vi "Ballard - 1553 - Raw Data Word Channel.vi"(8 "error in (no error)":errorcluster, 11 "Node Ptr":T1 format="%.0x") -> (0 "error out":errorcluster)   [LabVIEW 2017, in "Ballard 1553 System Explorer.lvlib"]
uses:
  Ballard 1553 System Explorer.lvlib
  <vilib>/NI Veristand/Custom Device API/Custom Device Item Ref.ctl
  <vilib>/NI VeriStand/Custom Device API/Custom Device API.lvlib
panel:
  out "Raw Data Default Value":u16 format="%.0x"
  in  "Header":cluster{"Section Name":string}={"Section Name"="Ballard - MIL-STD-1553 - Custom Device - Raw Data Word Channel"}
  in  "Description":string
  in  "Name":string
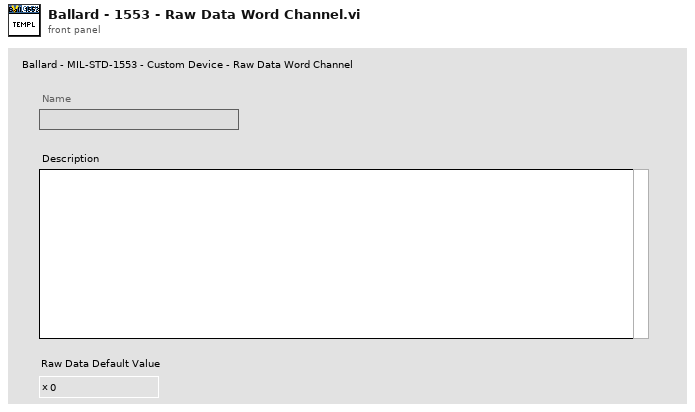
[diagram p1: front panel]
types:
  T1 = typedef "Custom Device API.lvlib/Custom Device Item Ref.ctl" = u64
  T2 = typedef "Custom Device API.lvlib/Custom Device Channel.ctl" = cluster{"Type":T3, "Units":string, "Default Value":dbl, "Faultable":bool, "Scalable":bool}
  T3 = typedef "Custom Device API.lvlib/Custom Device Channel Type.ctl" = enum16{"Input", "Output"}
  T4 = typedef "Custom Device API.lvlib/Custom Device Item Info.ctl" = cluster{"Name":string, "Is Channel":bool, "GUID":string, "Is Waveform":bool}
  T5 = typedef "Custom Device API.lvlib/Custom Device Commands.ctl" = enum16{"Default", "Item renamed", "Shutdown", "Dynamic button pressed"}
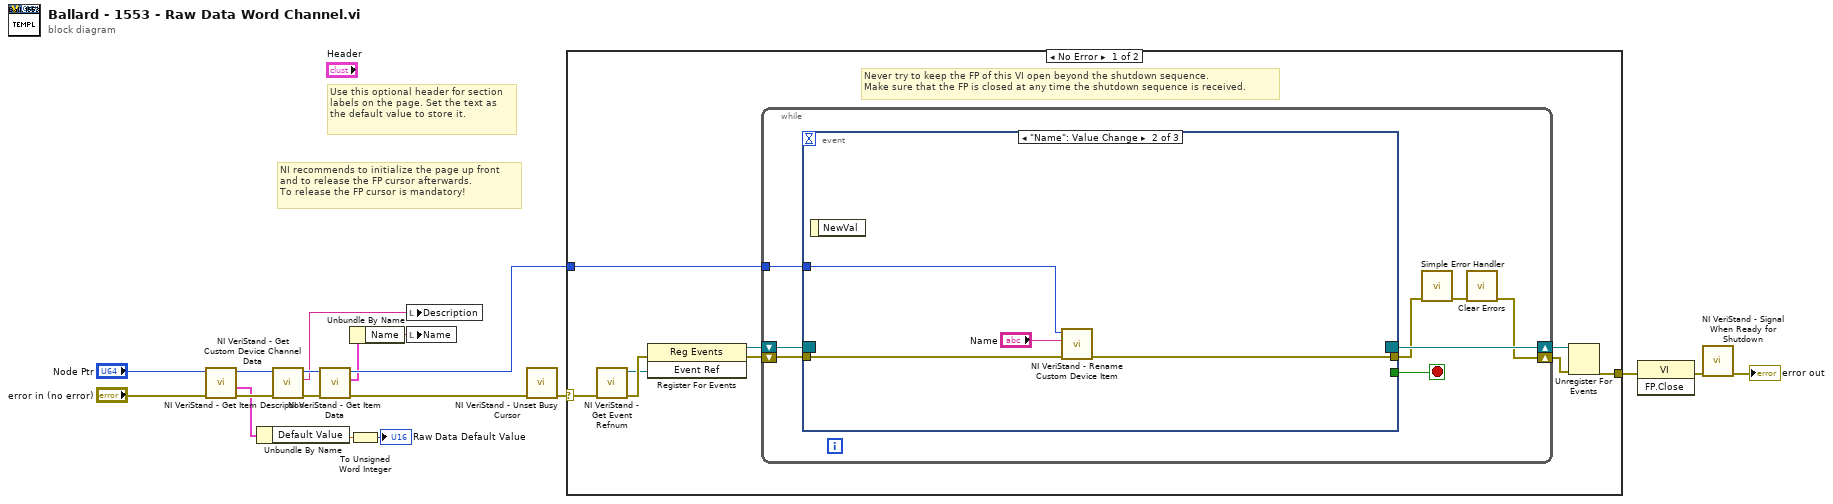
[diagram p0: block diagram]
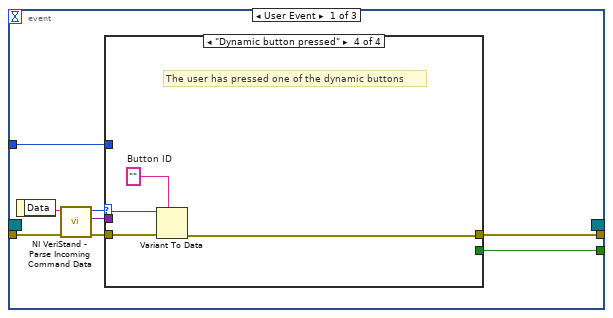
[diagram p2: hidden frame]
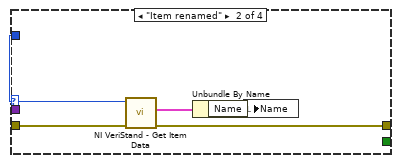
[diagram p4: hidden frame]
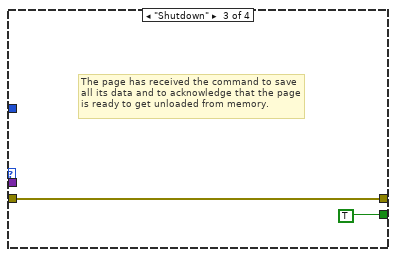
[diagram p5: hidden frame]
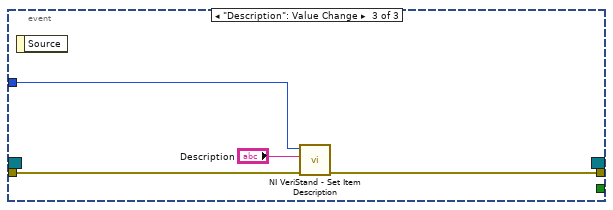
[diagram p6: hidden frame]
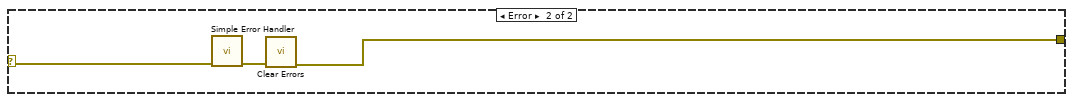
[diagram p7: hidden frame]
diagram:
  # "Use this optional header for section labels on the page. Set the text as the default value to store it."
  # "NI recommends to initialize the page up front\nand to release the FP cursor afterwards.\nTo release the FP cursor is mandatory!"
  n1 = call <vilib>:"NI VeriStand - Get Custom Device Channel Data.vi"("error in (no error)"="error in (no error)", "Channel Ref in"="Node Ptr") -> ("error out"=w5:errorcluster, "Channel"=w3:T2, "Channel Ref out"=w4:T1)  [unwired: 4 in, 3 out]
  n2 = Unbundle By Name(w3) -> ("Default Value"=w2:dbl)
  n3 = call <vilib>:"NI VeriStand - Get Item Description.vi"("error in (no error)"=w5, "Item Ref in"=w4) -> ("error out"=w10:errorcluster, "Description"=w11:string, "Item Ref out"=w12:T1)  [unwired: 7 out]
  n4 = call <vilib>:"NI VeriStand - Get Item Data.vi"("error in (no error)"=w10, "Item Ref in"=w12) -> ("error out"=w15:errorcluster, "Item Info"=w9:T4, "Item Ref out"=w13:T1)  [unwired: 7 out]
  n5 = Unbundle By Name(w9) -> ("Name"=w8:string)
  n6 = To Unsigned Word Integer(number=w2) -> (unsigned 16bit integer=→"Raw Data Default Value":u16)
  n7 = local write "Description"(w11) -> ()
  n8 = local write "Name"(w8) -> ()
  n9 = call <vilib>:"NI VeriStand - Unset Busy Cursor.vi"("error in (no error)"=w15) -> ("error out"=w14:errorcluster)  [unwired: 10 out]
  n10 = case shown="No Error" w14 {
    selector: w14 -> [w19 w66]
    tunnel: [w24 w64] -> w18
    tunnel: w13 -> [w20 _]
    frame No Error {
      # "Never try to keep the FP of this VI open beyond the shutdown sequence.\nMake sure that the FP is closed at any time the shutdown sequence is received."
      n11 = call <vilib>:"NI VeriStand - Get Event Refnum.vi"("error in (no error)"=w19) -> ("error out"=w27:errorcluster, "Event Ref"=w23:refnum<user-event>)  [unwired: 9 out]
      n12 = register-events(error in=w27, w23) -> (reference out=w21:refnum<event-registration>, error out=w22:errorcluster)  [unwired: 1 in]
      n13 = while {
        tunnel: w20 -> [w31]
        shift-right: [w28] -> w25
        shift-left: w22 -> [w34]
        shift-right: [w35] -> w26
        shift-left: w21 -> [w33]
        stop <- w32 stop-if-true
        n14 = event shown="[1] \"Name\": Value Change" {
          selector: w33 -> [_ _ _]
          dyn-events: [_ _ _] -> w35
          timeout: _ -> [_ _ _]
          tunnel: w34 -> [w43 w59 w62]
          tunnel: [w39 _ _] -> w32
          tunnel: [w38 w58 w61] -> w30
          tunnel: w31 -> [w37 w57 w63]
          event User Event {
            n15 = event-data() -> ("Data"=w42:string)  [unwired: 1 out]
            n16 = call <vilib>:"NI VeriStand - Parse Incoming Command Data.vi"("error in (no error)"=w43, "Incoming data"=w42) -> ("error out"=w41:errorcluster, "Outgoing data"=w36:variant, "Action"=w40:T5)  [unwired: 7 out]
            n17 = case shown="\"Dynamic button pressed\"" w40 {
              tunnel: w41 -> [w44 w49 w50 w55]
              tunnel: [_ _ TRUE _] -> w39
              tunnel: [w44 w46 w50 w52] -> w38
              tunnel: w37 -> [_ w48 _ _]
              tunnel: w36 -> [_ _ _ w54]
              frame "Default", Default {
              }
              frame "Item renamed" {
                n18 = call <vilib>:"NI VeriStand - Get Item Data.vi"("error in (no error)"=w49, "Item Ref in"=w48) -> ("error out"=w46:errorcluster, "Item Info"=w47:T4)  [unwired: 8 out]
                n19 = Unbundle By Name(w47) -> ("Name"=w45:string)
                n20 = local write "Name"(w45) -> ()
              }
              frame "Shutdown" {
                # "The page has received the command to save all its data and to acknowledge that the page is ready to get unloaded from memory."
              }
              frame "Dynamic button pressed" {
                w53 = ""  # Button ID
                # "The user has pressed one of the dynamic buttons"
                n21 = Variant To Data(error in=w55, type=w53, Variant=w54) -> (error out=w52:errorcluster)  [unwired: 1 out]
              }
            }
          }
          event "Name": Value Change {
            n22 = event-data() -> ()  [unwired: 2 out]
            n23 = call <vilib>:"NI VeriStand - Rename Custom Device Item.vi"("error in (no error)"=w59, "New Name"="Name", "Item Ref in"=w57) -> ("error out"=w58:errorcluster)  [unwired: 1 in, 7 out]
          }
          event "Description": Value Change {
            n24 = event-data() -> ()  [unwired: 2 out]
            n25 = call <vilib>:"NI VeriStand - Set Item Description.vi"("error in (no error)"=w62, "Description"="Description", "Item Ref in"=w63) -> ("error out"=w61:errorcluster)  [unwired: 8 out]
          }
        }
        n26 = call <vilib>:"Simple Error Handler.vi"("error in (no error)"=w30) -> ("error out"=w29:errorcluster)  [unwired: 1 in, 7 out]
        n27 = call <vilib>:"Clear Errors.vi"("error in (no error)"=w29) -> ("error out"=w28:errorcluster)  [unwired: 1 in, 5 out]
      }
      n28 = Unregister For Events(event registration refnum=w26, error in=w25) -> (error out=w24:errorcluster)
    }
    frame Error {
      n29 = call <vilib>:"Simple Error Handler.vi"("error in (no error)"=w66) -> ("error out"=w65:errorcluster)  [unwired: 1 in, 7 out]
      n30 = call <vilib>:"Clear Errors.vi"("error in (no error)"=w65) -> ("error out"=w64:errorcluster)  [unwired: 1 in, 5 out]
    }
  }
  n31 = invoke class="VI" method="FP.Close"(error in=w18) -> (error out=w17:errorcluster)  [unwired: 2 in, 2 out]
  n32 = call <vilib>:"NI VeriStand - Signal When Ready for Shutdown.vi"("error in (no error)"=w17) -> ("error out"=→"error out":errorcluster)  [unwired: 10 out]
